vi "SW_get_config_of_Zones_and_IO.vi"(0 "Sync parameters cluster input":T2={"SYNC configuration"=12, "IO 1 configuration"=1, "IO 2 configuration"=1, "IO 3 configuration"=0, "IO 4 configuration"=0, "Activate ext. RS-232"=0, "IO inversion config."=0}) -> (1 "Zones out config":u32, 2 "Zones out config bin":bool[](array[boolean]), 3 "Ports IO config (OUT is FALSE)":bool[](array[boolean]), 4 "IO inversion config.":u16)   [LabVIEW 2016]
uses:
  <vilib>/Utility/miscctls.llb/LVPointTypeDef.ctl
panel:
  out "IO status indicator":T1
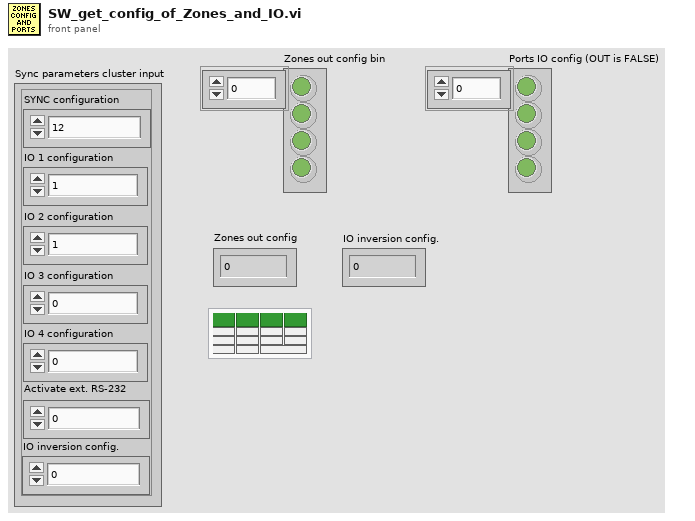
[diagram p1: front panel]
types:
  T1 = cluster{"IO1":bool, "IO2":bool, "IO3":bool, "IO4":bool, "Z1":bool, "Z2":bool, "Z3":bool, "Z4":bool, "St1":bool, "St2":bool, "St3":bool, "St4":bool, "Syn1":bool, "Syn2":bool, "RS-232 ext. activated":bool}
  T2 = cluster{"SYNC configuration":u16, "IO 1 configuration":u16, "IO 2 configuration":u16, "IO 3 configuration":u16, "IO 4 configuration":u16, "Activate ext. RS-232":u16, "IO inversion config.":u16}
  T3 = typedef "LVPointTypeDef.ctl" = cluster{"Horizontal":i16, "Vertical":i16}
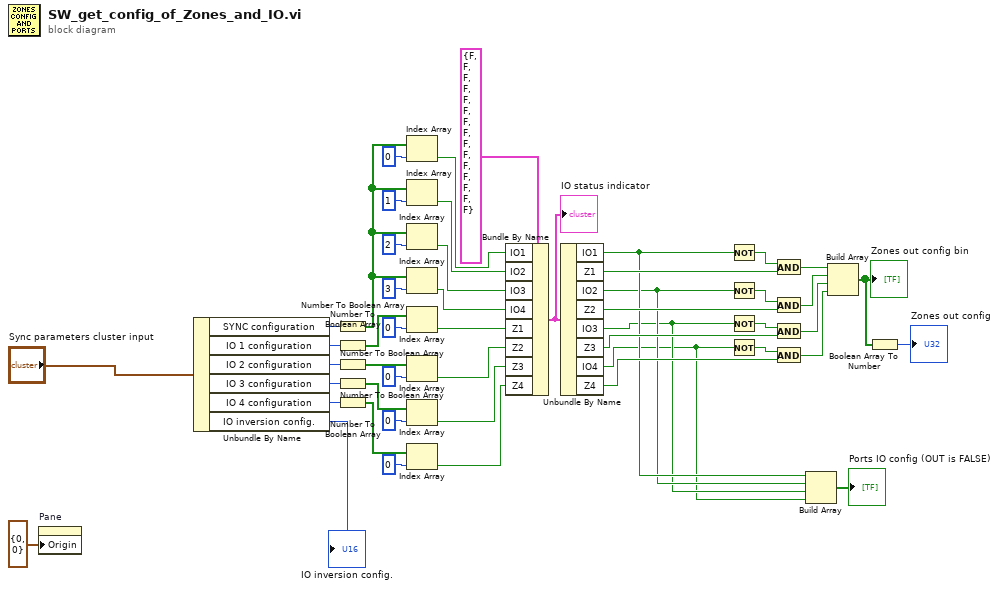
[diagram p0: block diagram]
diagram:
  n1 = property on="Pane" class="Pane"("Origin"=T3 {"Horizontal"=0, "Vertical"=0}) -> ()  [unwired: 2 in, 2 out]
  n2 = Unbundle By Name("Sync parameters cluster input") -> ("SYNC configuration"=w45:u16, "IO 1 configuration"=w39:u16, "IO 2 configuration"=w34:u16, "IO 3 configuration"=w31:u16, "IO 4 configuration"=w30:u16, "IO inversion config."=→"IO inversion config.":u16)
  n3 = Number To Boolean Array(number=w45) -> (Boolean array=w44:bool[])
  n4 = Number To Boolean Array(number=w39) -> (Boolean array=w38:bool[])
  n5 = Number To Boolean Array(number=w34) -> (Boolean array=w35:bool[])
  n6 = Number To Boolean Array(number=w31) -> (Boolean array=w33:bool[])
  n7 = Number To Boolean Array(number=w30) -> (Boolean array=w32:bool[])
  n8 = Index Array(array=w44, index=0) -> (element=w49:bool)
  n9 = Index Array(array=w44, index=1) -> (element=w48:bool)
  n10 = Index Array(array=w44, index=2) -> (element=w47:bool)
  n11 = Index Array(array=w44, index=3) -> (element=w46:bool)
  n12 = Index Array(array=w38, index=0) -> (element=w25:bool)
  n13 = Index Array(array=w35, index=0) -> (element=w24:bool)
  n14 = Index Array(array=w33, index=0) -> (element=w23:bool)
  n15 = Index Array(array=w32, index=0) -> (element=w22:bool)
  n16 = Bundle By Name(cluster=T1 {"IO1"=FALSE, "IO2"=FALSE, "IO3"=FALSE, "IO4"=FALSE, "Z1"=FALSE, "Z2"=FALSE, "Z3"=FALSE, "Z4"=FALSE, "St1"=FALSE, "St2"=FALSE, "St3"=FALSE, "St4"=FALSE, "Syn1"=FALSE, "Syn2"=FALSE, "RS-232 ext. activated"=FALSE} ("IO status indicator 2"), "IO1"=w49, "IO2"=w48, "IO3"=w47, "IO4"=w46, "Z1"=w25, "Z2"=w24, "Z3"=w23, "Z4"=w22) -> (w13:T1)
  "IO status indicator" <- w13
  n17 = Unbundle By Name(w13) -> ("IO1"=w5:bool, "Z1"=w10:bool, "IO2"=w4:bool, "Z2"=w9:bool, "IO3"=w3:bool, "Z3"=w8:bool, "IO4"=w2:bool, "Z4"=w7:bool)
  n18 = Not(x=w5) -> (.not. x?=w21:bool)
  n19 = Not(x=w4) -> (.not. x?=w20:bool)
  n20 = Not(x=w3) -> (.not. x?=w19:bool)
  n21 = Not(x=w2) -> (.not. x?=w18:bool)
  n22 = And(x=w21, y=w10) -> (x .and. y?=w17:bool)
  n23 = And(x=w20, y=w9) -> (x .and. y?=w16:bool)
  n24 = And(x=w19, y=w8) -> (x .and. y?=w15:bool)
  n25 = And(x=w18, y=w7) -> (x .and. y?=w14:bool)
  n26 = Build Array(w5, w4, w3, w2) -> (→"Ports IO config (OUT is FALSE)":bool[])
  n27 = Build Array(w17, w16, w15, w14) -> (w12:bool[])
  "Zones out config bin" <- w12
  n28 = Boolean Array To Number(Boolean array=w12) -> (number=→"Zones out config":u32)
